vi "Read model_name.vi"(8 "error in (no error)":errorcluster, 11 "llm_openai_chatmodels in":refnum<class "llm_gemini_chatmodels.lvclass">) -> (0 "error out":errorcluster, 2 "model_name":string(combo), 3 "llm_openai_chatmodels out":refnum<class "llm_gemini_chatmodels.lvclass">)   [LabVIEW 2020, in "llm_gemini_chatmodels.lvclass"]
uses:
  llm_gemini_chatmodels.lvclass
  llm_gemini_chatmodels.lvclass/llm_gemini_chatmodels.ctl
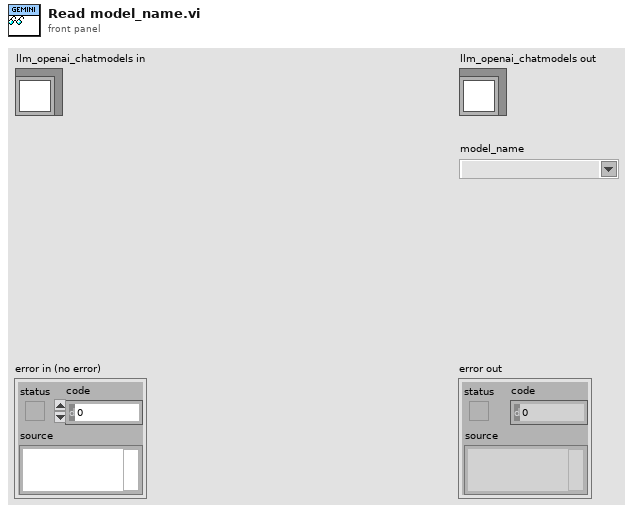
[diagram p1: front panel]
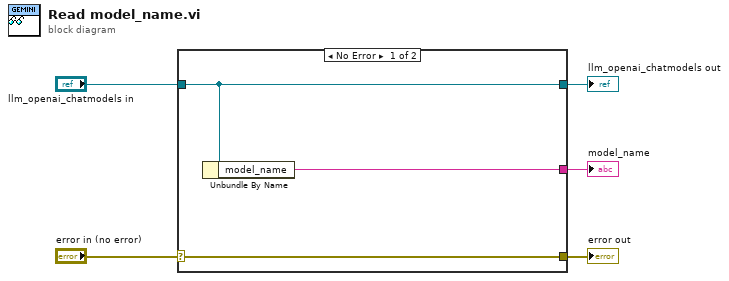
[diagram p0: block diagram]
diagram:
  n1 = case shown="No Error" "error in (no error)" {
    selector: "error in (no error)" -> [w8 w9]
    tunnel: [w8 w9] -> w4
    tunnel: [w7 w10] -> w2
    tunnel: "llm_openai_chatmodels in" -> [w7 w10]
    tunnel: [w6 _] -> w1
    frame No Error {
      n2 = Unbundle By Name(w7) -> ("model_name"=w6:string)
    }
    frame Error {
    }
  }
  "error out" <- w4
  "llm_openai_chatmodels out" <- w2
  "model_name" <- w1
